vi "Create Measurement Client.vi"() -> ()   [LabVIEW 2021, in "MeasurementClient Editor.lvlib"]
uses:
  _MeasurementClient Utility/MeasurementClient Editor.lvlib
  <vilib>/Utility/error.llb/ErrWarn.ctl
  <vilib>/gRPC/Generated APIs/ni/measurementlink/discovery/v1/RPC Messages/ni_measurementlink_discovery_v1_EnumerateServicesRequest.ctl
  _Generator Helpers/Generator Helpers.lvlib
  <vilib>/gRPC/Generated APIs/ni/measurementlink/discovery/v1/ni.measurementlink.discovery.v1.api.lvlib
  <vilib>/Plug-In SDKs/Clients/Discovery V1/NI Discovery V1 Client.lvlib
panel:
  in  "Tab Control":enum32{"Inputs", "Status"}(tab)
  out "Active Project Name":string
  in  "Available Measurements":i32(listbox)=-1
  in  "Create Client":bool
  out "Warning":T1 caption="Measurement plug-in client name must be unique and cannot contain any of the following characters:\n           \\ / : * ? \" < > |"
  out "Error Message":string
  in  "Client Status":i32(listbox)=-1 caption="Measurement Plug-In Client Creation Status"
  # "* Project in which the measurement plug-in client vi will be created"
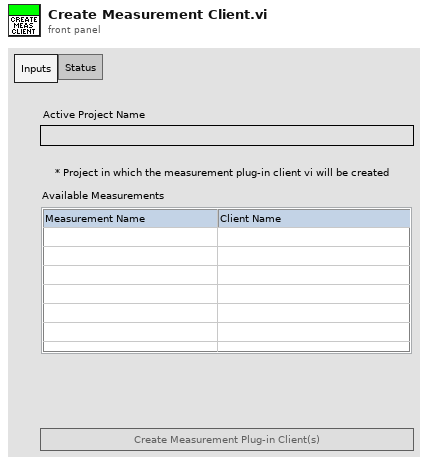
[diagram p1: front panel]
types:
  T1 = typedef "ErrWarn.ctl" = bool
  T2 = enum8{"Enabled", "Disabled", "Disabled and Grayed Out"}
  T3 = typedef "ni.measurementlink.discovery.v1.api.lvlib/ni_measurementlink_discovery_v1_EnumerateServicesRequest.ctl" = cluster{"provided_interface":string}
  T4 = typedef "ni.measurementlink.discovery.v1.api.lvlib/ni_measurementlink_discovery_v1_EnumerateServicesResponse.ctl" = cluster{"available_services":T5[]}
  T5 = typedef "ni.measurementlink.discovery.v1.api.lvlib/ni_measurementlink_discovery_v1_ServiceDescriptor.ctl" = cluster{"display_name":string, "description_url":string, "provided_interfaces":string[], "service_class":string, "annotations":T6[]}
  T6 = typedef "ni.measurementlink.discovery.v1.api.lvlib/ni_measurementlink_discovery_v1_ServiceDescriptor_AnnotationsEntry.ctl" = cluster{"key":string, "value":string}
  T7 = cluster{"project ref":refnum<vi>, "multicolumnListbox ref":refnum<vi>, "available measurement details":T4, "statusListbox ref":refnum<vi>, "error messages":string[]}
  T8 = typedef "ni.measurementlink.measurement.v2.api.lvlib/Measurement Service Client.lvlib/ni_measurementlink_measurement_v2_Output.ctl" = cluster{"field_number":i32, "type":T9, "name":string, "repeated":bool, "annotations":T10[], "message_type":string}
  T9 = typedef "ni.measurementlink.measurement.v2.api.lvlib/Measurement Service Client.lvlib/google_protobuf_Field_Kind.ctl" = enum32{"TYPE_UNKNOWN", "TYPE_DOUBLE", "TYPE_FLOAT", "TYPE_INT64", "TYPE_UINT64", "TYPE_INT32", "TYPE_FIXED64", "TYPE_FIXED32", "TYPE_BOOL", "TYPE_STRING", "TYPE_GROUP", "TYPE_MESSAGE", "TYPE_BYTES", "TYPE_UINT32", "TYPE_ENUM", "TYPE_SFIXED32", "TYPE_SFIXED64", "TYPE_SINT32", "TYPE_SINT64"}
  T10 = typedef "ni.measurementlink.measurement.v2.api.lvlib/Measurement Service Client.lvlib/ni_measurementlink_measurement_v2_Output_AnnotationsEntry.ctl" = cluster{"key":string, "value":string}
  T11 = typedef "ni.measurementlink.measurement.v2.api.lvlib/Measurement Service Client.lvlib/ni_measurementlink_measurement_v2_ConfigurationParameter.ctl" = cluster{"field_number":i32, "type":T9, "name":string, "repeated":bool, "annotations":T12[], "message_type":string}
  T12 = typedef "ni.measurementlink.measurement.v2.api.lvlib/Measurement Service Client.lvlib/ni_measurementlink_measurement_v2_ConfigurationParameter_AnnotationsEntry.ctl" = cluster{"key":string, "value":string}
  T13 = typedef "LVPoint32TypeDef.ctl" = cluster{"Horizontal":i32, "Vertical":i32}
  T14 = typedef "LVRowAndColumnTypeDef.ctl" = cluster{"Row":i32, "Column":i32}
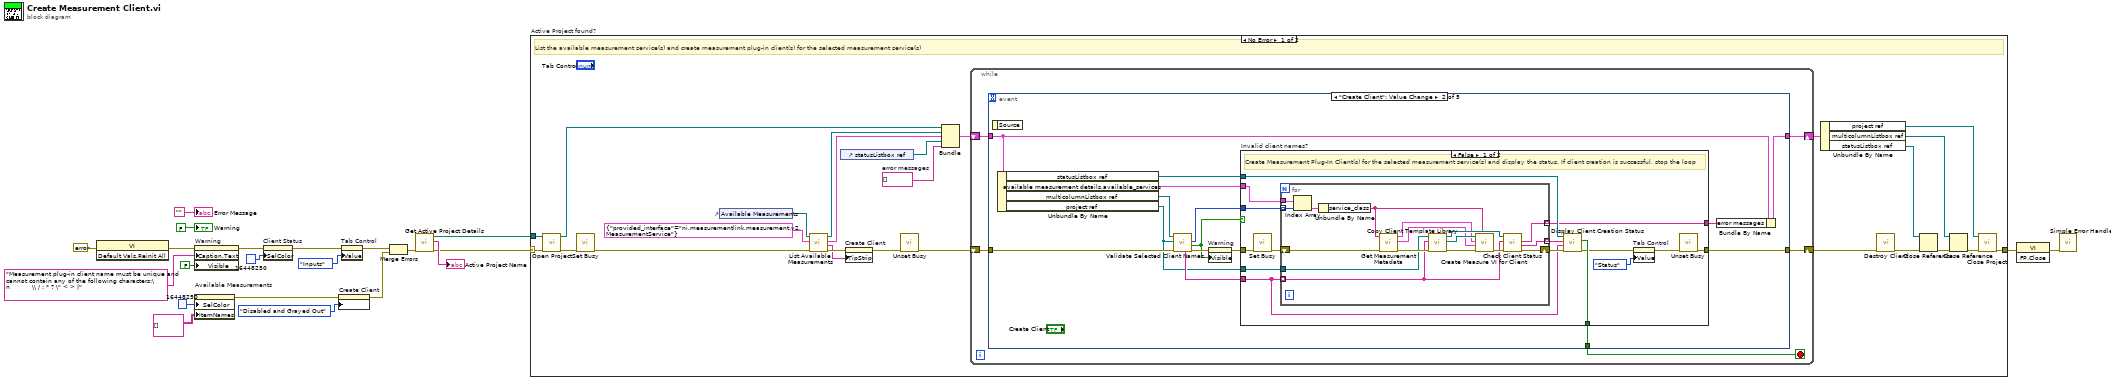
[diagram p0: block diagram]
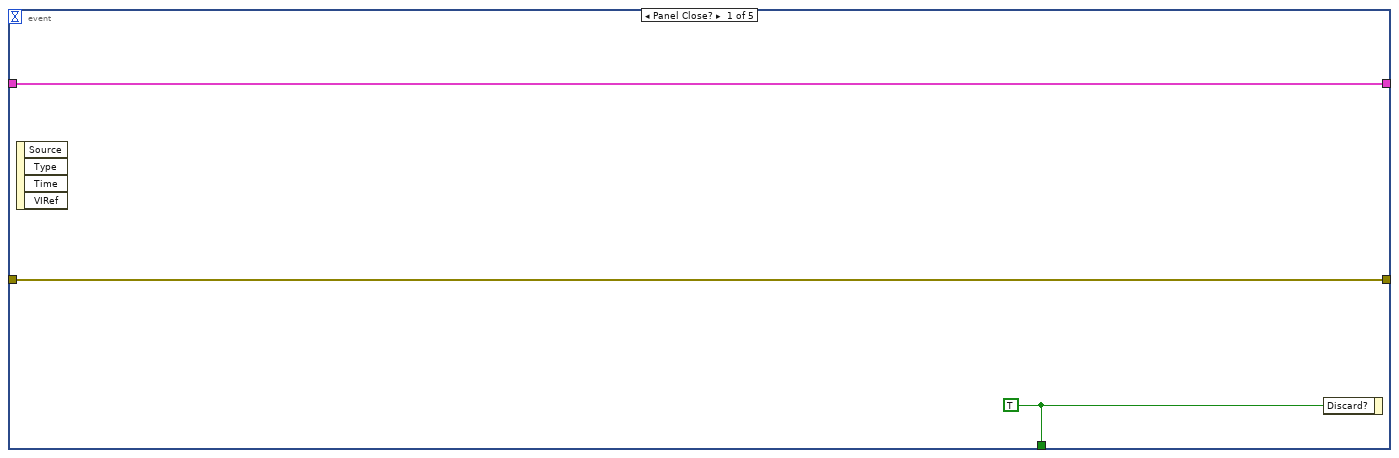
[diagram p2: hidden frame]
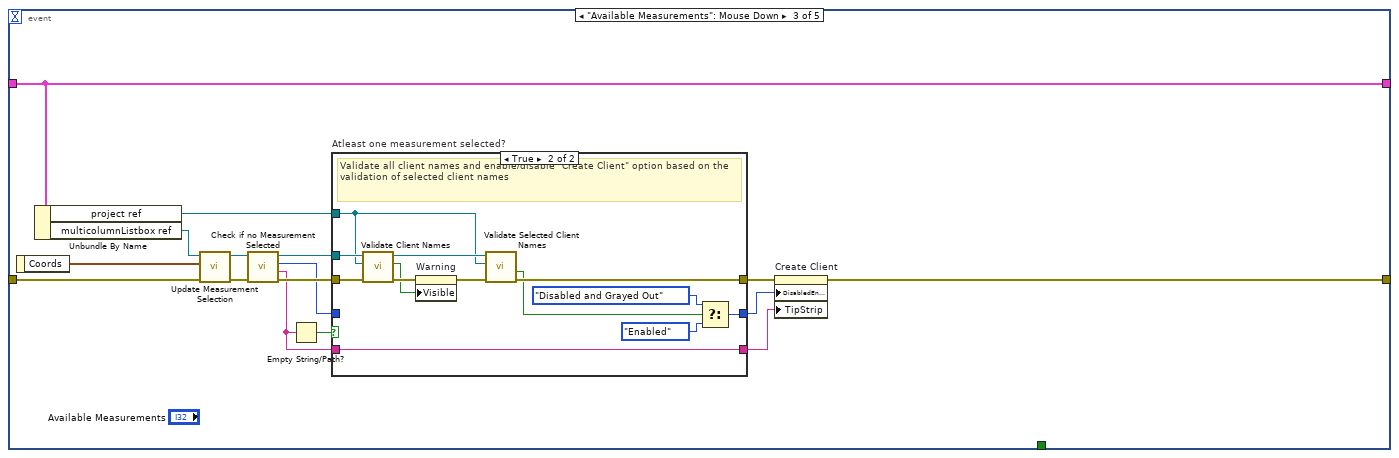
[diagram p4: hidden frame]
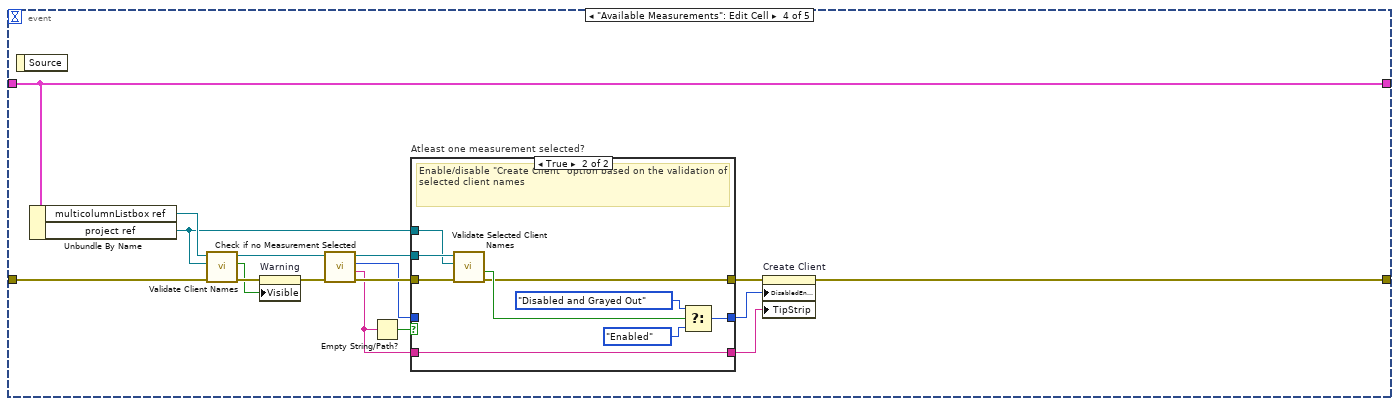
[diagram p6: hidden frame]
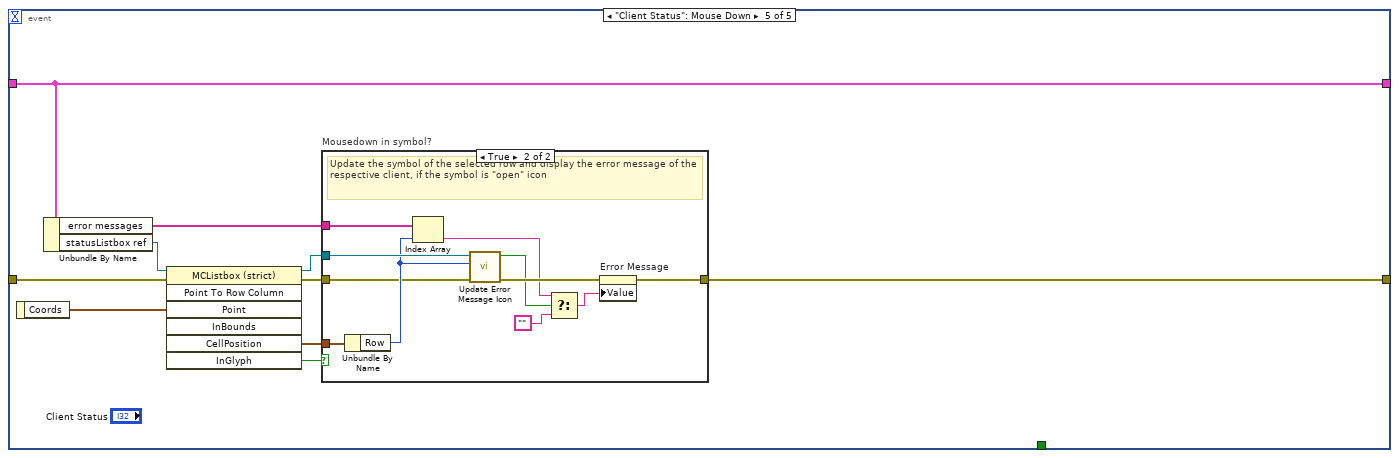
[diagram p8: hidden frame]
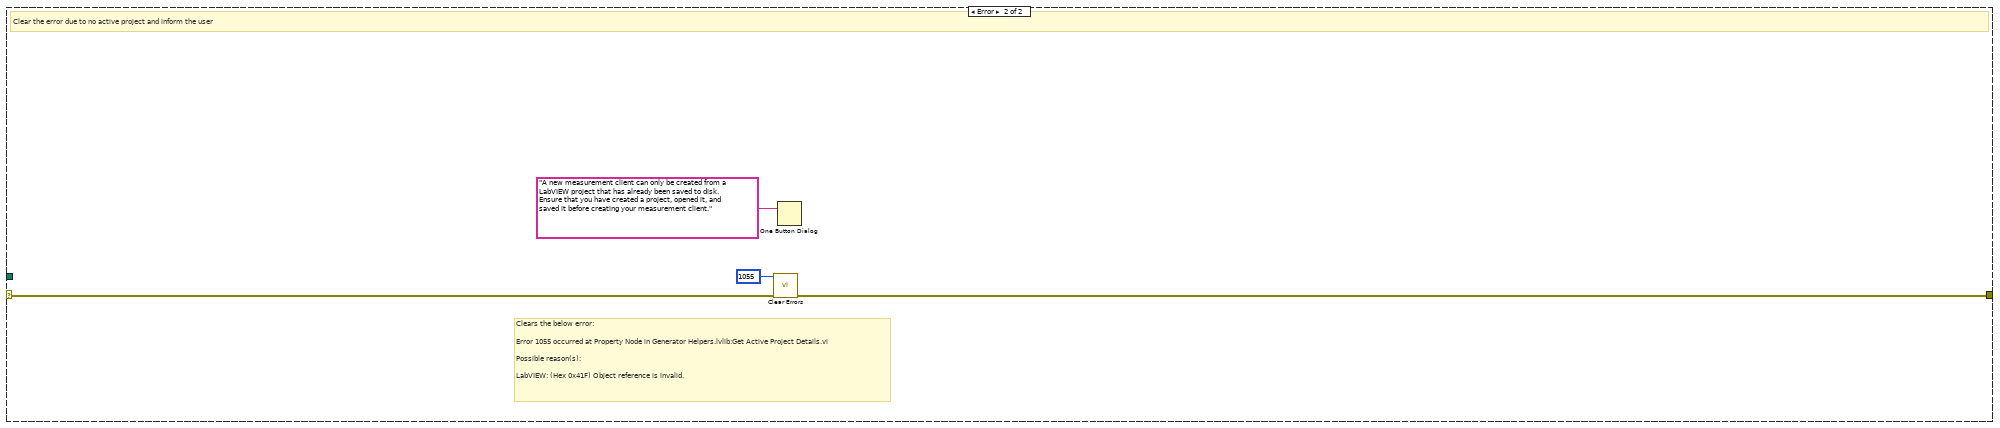
[diagram p10: hidden frame]
diagram:
  n1 = invoke class="VI" method="Default Vals.Reinit All"(error in=errorcluster {"status"=FALSE, "code"=0, "source"=""} ("error in (no error)")) -> (error out=w16:errorcluster)  [unwired: 2 in, 2 out]
  n2 = property on="Warning" class="Bool"(error in=w16, "Caption.Text"="Measurement plug-in client name must be unique and cannot contain any of the following characters:\n           \\ / : * ? \" < > |" ("Status"), "Visible"=FALSE) -> (error out=w6:errorcluster)  [unwired: 1 in, 1 out]
  n3 = property on="Available Measurements" class="MCListbox (strict)"("SelColor"=u32 16448250 ("Selection Color"), "ItemNames"=string[][] [] ("Item Names")) -> (error out=w3:errorcluster)  [unwired: 2 in, 1 out]
  n4 = property on="Client Status" class="MCListbox (strict)"(error in=w6, "SelColor"=u32 16448250 ("Selection Color")) -> (error out=w7:errorcluster)  [unwired: 1 in, 1 out]
  n5 = property on="Create Client" class="Bool"(error in=w3, "DisabledEnum"=T2."Disabled and Grayed Out" ("Disabled")) -> (error out=w2:errorcluster)  [unwired: 1 in, 1 out]
  n6 = property on="Tab Control" class="TabCtl (strict)"(error in=w7, "Value"=enum32{"Inputs", "Status"}."Inputs" ("Tab Control")) -> (error out=w5:errorcluster)  [unwired: 1 in, 1 out]
  n7 = Merge Errors(w5, w2) -> (w1:errorcluster)
  n8 = call "Get Active Project Details.vi"("error in"=w1) -> ("error out"=w11:errorcluster, "name"=→"Active Project Name":string, "path"=w15:path)  [unwired: 8 in]
  n9 = case "Active Project found?" shown="No Error" w11 {
    selector: w11 -> [w37 w187]
    tunnel: [w31 w190] -> w20
    tunnel: w15 -> [w47 _]
    frame No Error {
      w30 = string[] []  # error messages
      # "List the available measurement service(s) and create measurement plug-in client(s) for the selected measurement service(s)"
      n10 = call "Open Project.vi"("error in"=w37, "path"=w47) -> ("error out"=w38:errorcluster, "project ref"=w35:refnum<vi>)  [unwired: 8 in]
      n11 = call <vilib>:"Set Busy.vi"("error in (no error)"=w38) -> ("error out"=w40:errorcluster)  [unwired: 9 in, 1 out]
      n12 = control-ref of="Available Measurements"() -> (w43:refnum<vi>)
      n13 = call "List Available Measurements.vi"("error in (no error)"=w40, "enumerate services request"=T3 {"provided_interface"="ni.measurementlink.measurement.v2.MeasurementService"} ("request data"), "multicolumnListbox ref in"=w43) -> ("error out"=w42:errorcluster, "warning"=w24:string, "available measurement details"=w46:T4, "multicolumnListbox ref"=w27:refnum<vi>)  [unwired: 5 in]
      n14 = control-ref of="statusListbox ref"() -> (w23:refnum<vi>)
      n15 = property on="Create Client" class="Bool"(error in=w42, "TipStrip"=w24) -> (error out=w41:errorcluster)  [unwired: 1 in, 1 out]
      n16 = call <vilib>:"Unset Busy.vi"("error in (no error)"=w41) -> ("error out"=w39:errorcluster)  [unwired: 10 in]
      n17 = Bundle("project ref"=w35, "multicolumnListbox ref"=w27, "available measurement details"=w46, "statusListbox ref"=w23, "error messages"=w30) -> (w25:T7)  [unwired: 1 in]
      n18 = while {
        shift-right: [w51] -> w44
        shift-left: w39 -> [w52]
        shift-right: [w49] -> w26
        shift-left: w25 -> [w50]
        stop <- w48 stop-if-true
        n19 = event shown="[1] \"Create Client\": Value Change" {
          selector: _ -> [_ _ _ _ _]
          dyn-events: _ -> [_ _ _ _ _]
          timeout: _ -> [_ _ _ _ _]
          tunnel: w52 -> [w55 w70 w114 w151 w171]
          tunnel: [w55 w57 w113 w147 w174] -> w51
          tunnel: w50 -> [w54 w65 w119 w152 w172]
          tunnel: [w54 w61 w119 w152 w172] -> w49
          tunnel: [w53 w58 _ _ _] -> w48
          event Panel Close? {
            w53 = TRUE ("Discard?")
            # "Discard panel close and stop the execution of measurement plug-in client generator"
            n20 = event-data() -> ()  [unwired: 1 in, 4 out]
            n21 = event-data("Discard?"=w53) -> ()  [unwired: 1 in, 1 out]
          }
          event "Create Client": Value Change {
            # "Validate client name and create measurement plug-in client for the selected measurement service(s), if no invalid client name"
            n22 = event-data() -> ()  [unwired: 1 in, 1 out]
            n23 = Unbundle By Name(w65) -> ("statusListbox ref"=w62:refnum<vi>, "available measurement details.available_services"=w60:T5[], "multicolumnListbox ref"=w69:refnum<vi>, "project ref"=w63:refnum<vi>)
            n24 = call "Validate Selected Client Names.vi"("error in (no error)"=w70, "project ref"=w63, "multicolumnListbox in"=w69) -> ("error out"=w68:errorcluster, "warning?"=w59:bool, "selected measurement indices"=w66:i32[], "selected client names"=w64:string[])  [unwired: 4 in, 1 out]
            n25 = property on="Warning" class="Bool"(error in=w68, "Visible"=w59) -> (error out=w67:errorcluster)  [unwired: 1 in, 1 out]
            n26 = case "Invalid client names?" shown="False" w59 {
              tunnel: w67 -> [w85 w103]
              tunnel: w66 -> [w84 _]
              tunnel: w64 -> [w77 _]
              tunnel: w63 -> [w79 _]
              tunnel: [w72 w103] -> w57
              tunnel: w62 -> [w80 _]
              tunnel: w60 -> [w78 _]
              tunnel: [w76 _] -> w58
              tunnel: [w71 _] -> w56
              frame False {
                # "Create Measurement Plug-In Client(s) for the selected measurement service(s) and display the status. If client creation is successful, stop the loop"
                n27 = call <vilib>:"Set Busy.vi"("error in (no error)"=w85) -> ("error out"=w83:errorcluster)  [unwired: 9 in, 1 out]
                n28 = for {
                  tunnel: w78 -> [w100]
                  tunnel: w77 -> [w92] mode=indexing
                  shift-right: [w97] -> w82
                  shift-left: w83 -> [w94]
                  tunnel: w84 -> [w93] mode=indexing
                  tunnel: [w91] -> w81 mode=indexing
                  tunnel: w79 -> [w90]
                  tunnel: [w88] -> w71 mode=indexing
                  n29 = Index Array(array=w100, index=w93) -> (element=w99:T5)
                  n30 = Unbundle By Name(w99) -> ("service_class"=w89:string)
                  n31 = call "Get Measurement Metadata.vi"("error in"=w94, "service_class"=w89) -> ("error out"=w101:errorcluster, "outputs"=w86:T8[], "configuration_parameters"=w87:T11[])  [unwired: 7 in]
                  n32 = call "Copy Client Template Library.vi"("error in"=w101, "client name"=w92, "project ref"=w90) -> ("error out"=w102:errorcluster, "measure vi refnum"=w98:refnum<vi>, "project ref out"=w95:refnum<vi>)  [unwired: 6 in]
                  n33 = call "Create Measure VI for Client.vi"("client service_class"=w89, "error in"=w102, "results data"=w86, "configuration data"=w87, "measure vi refnum"=w98) -> ("error out"=w96:errorcluster)  [unwired: 6 in]
                  n34 = call "Check Client Status.vi"("error in"=w96, "client name"=w92, "project ref in"=w95) -> ("error out"=w97:errorcluster, "status"=w91:string, "error message"=w88:string)  [unwired: 5 in, 1 out]
                }
                n35 = call "Display Client Creation Status.vi"("error in"=w82, "client names"=w77, "status"=w81, "statusListbox in"=w80) -> ("error out"=w74:errorcluster, "all success?"=w76:bool)  [unwired: 5 in, 1 out]
                n36 = property on="Tab Control" class="TabCtl (strict)"(error in=w74, "Value"=enum32{"Inputs", "Status"}."Status" ("Tab Control")) -> (error out=w73:errorcluster)  [unwired: 1 in, 1 out]
                n37 = call <vilib>:"Unset Busy.vi"("error in (no error)"=w73) -> ("error out"=w72:errorcluster)  [unwired: 10 in]
              }
              frame True {
                # "Pass"
              }
            }
            n38 = Bundle By Name(cluster=w65, "error messages"=w56) -> (w61:T7)
          }
          event "Available Measurements": Mouse Down {
            # "Update the selection of measurement service and enable/disable \"Create Client\" accordingly"
            n39 = event-data() -> ("Coords"=w112:T13)  [unwired: 1 in]
            n40 = Unbundle By Name(w119) -> ("project ref"=w104:refnum<vi>, "multicolumnListbox ref"=w118:refnum<vi>)
            n41 = call "Update Measurement Selection.vi"("error in (no error)"=w114, "mouseDown coords"=w112, "multicolumnListbox in"=w118) -> ("error out"=w116:errorcluster, "multicolumnListbox out"=w117:refnum<vi>)  [unwired: 7 in]
            n42 = call "Check if no Measurement Selected.vi"("error in (no error)"=w116, "multicolumnListbox in"=w117) -> ("error out"=w115:errorcluster, "warning?"=w105:string, "create client disabled?"=w107:T2, "multicolumnListbox out"=w110:refnum<vi>)  [unwired: 6 in]
            n43 = Empty String/Path?(string/path=w105) -> (empty?=w109:bool)
            n44 = case "Atleast one measurement selected?" shown="True" w109 {
              tunnel: w115 -> [w122 w127]
              tunnel: [w122 w131] -> w111
              tunnel: w110 -> [_ w126]
              tunnel: [w121 w132] -> w106
              tunnel: w105 -> [w121 w132]
              tunnel: [w120 w133] -> w108
              tunnel: w107 -> [w120 _]
              tunnel: w104 -> [_ w123]
              frame False {
                # "Enable/disable the \"Create Client\" option based on measurement selection"
              }
              frame True {
                # "Validate all client names and enable/disable \"Create Client\" option based on the validation of selected client names"
                n45 = call "Validate Client Names.vi"("error in (no error)"=w127, "project ref"=w123, "multicolumnListbox in"=w126) -> ("error out"=w129:errorcluster, "warning?"=w128:bool, "multicolumnListbox out"=w125:refnum<vi>)  [unwired: 6 in]
                n46 = property on="Warning" class="Bool"(error in=w129, "Visible"=w128) -> (error out=w124:errorcluster)  [unwired: 1 in, 1 out]
                n47 = call "Validate Selected Client Names.vi"("error in (no error)"=w124, "project ref"=w123, "multicolumnListbox in"=w125) -> ("error out"=w131:errorcluster, "warning?"=w130:bool)  [unwired: 4 in, 3 out]
                n48 = Select(t=T2."Disabled and Grayed Out" ("Disabled"), s=w130, f=T2."Enabled") -> (s? t:f=w133:T2)
              }
            }
            n49 = property on="Create Client" class="Bool"(error in=w111, "DisabledEnum"=w108, "TipStrip"=w106) -> (error out=w113:errorcluster)  [unwired: 1 in, 1 out]
          }
          event "Available Measurements": Edit Cell {
            n50 = event-data() -> ()  [unwired: 1 in, 1 out]
            n51 = Unbundle By Name(w152) -> ("multicolumnListbox ref"=w148:refnum<vi>, "project ref"=w136:refnum<vi>)
            n52 = call "Validate Client Names.vi"("error in (no error)"=w151, "project ref"=w136, "multicolumnListbox in"=w148) -> ("error out"=w150:errorcluster, "warning?"=w149:bool, "multicolumnListbox out"=w143:refnum<vi>)  [unwired: 6 in]
            n53 = property on="Warning" class="Bool"(error in=w150, "Visible"=w149) -> (error out=w144:errorcluster)  [unwired: 1 in, 1 out]
            n54 = call "Check if no Measurement Selected.vi"("error in (no error)"=w144, "multicolumnListbox in"=w143) -> ("error out"=w141:errorcluster, "warning?"=w137:string, "create client disabled?"=w139:T2, "multicolumnListbox out"=w142:refnum<vi>)  [unwired: 6 in]
            n55 = Empty String/Path?(string/path=w137) -> (empty?=w140:bool)
            n56 = case "Atleast one measurement selected?" shown="True" w140 {
              tunnel: [w154 w163] -> w146
              tunnel: [w155 w160] -> w145
              tunnel: w142 -> [_ w159]
              tunnel: w141 -> [w154 w158]
              tunnel: w139 -> [w155 _]
              tunnel: [w153 w157] -> w138
              tunnel: w137 -> [w153 w157]
              tunnel: w136 -> [_ w156]
              frame False {
                # "Enable/disable the \"Create Client\" option based on measurement selection"
              }
              frame True {
                # "Enable/disable \"Create Client\" option based on the validation of selected client names"
                n57 = call "Validate Selected Client Names.vi"("error in (no error)"=w158, "project ref"=w156, "multicolumnListbox in"=w159) -> ("error out"=w163:errorcluster, "warning?"=w164:bool)  [unwired: 4 in, 3 out]
                n58 = Select(t=T2."Disabled and Grayed Out" ("Disabled"), s=w164, f=T2."Enabled") -> (s? t:f=w160:T2)
              }
            }
            n59 = property on="Create Client" class="Bool"(error in=w146, "DisabledEnum"=w145, "TipStrip"=w138) -> (error out=w147:errorcluster)  [unwired: 1 in, 1 out]
          }
          event "Client Status": Mouse Down {
            n60 = event-data() -> ("Coords"=w168:T13)  [unwired: 1 in]
            n61 = Unbundle By Name(w172) -> ("error messages"=w173:string[], "statusListbox ref"=w169:refnum<vi>)
            n62 = invoke class="MCListbox (strict)" method="Point To Row Column"(reference=w169, error in=w171, "Point"=w168) -> (reference out=w166:refnum<vi>, error out=w170:errorcluster, "CellPosition"=w167:T14, "InGlyph"=w165:bool)  [unwired: 4 in, 3 out]
            n63 = case "Mousedown in symbol?" shown="True" w165 {
              tunnel: [w175 w180] -> w174
              tunnel: w167 -> [_ w186]
              tunnel: w173 -> [_ w185]
              tunnel: w170 -> [w175 w182]
              tunnel: w166 -> [_ w184]
              frame False {
                # "Pass"
              }
              frame True {
                # "Update the symbol of the selected row and display the error message of the respective client, if the symbol is \"open\" icon"
                n64 = Unbundle By Name(w186) -> ("Row"=w183:i32)
                n65 = Index Array(array=w185, index=w183) -> (element=w178:string)
                n66 = call "Update Error Message Icon.vi"("error in"=w182, "selected row"=w183, "statusListbox in"=w184) -> ("error out"=w181:errorcluster, "open?"=w179:bool)  [unwired: 7 in]
                n67 = Select(t=w178, s=w179, f="") -> (s? t:f=w176:string)
                n68 = property on="Error Message" class="Str"(error in=w181, "Value"=w176) -> (error out=w180:errorcluster)  [unwired: 1 in, 1 out]
              }
            }
          }
        }
      }
      n69 = Unbundle By Name(w26) -> ("project ref"=w32:refnum<vi>, "multicolumnListbox ref"=w45:refnum<vi>, "statusListbox ref"=w28:refnum<vi>)
      n70 = call <vilib>:"Destroy Client.vi"("error in"=w44) -> ("error out"=w34:errorcluster)  [unwired: 10 in]
      n71 = Close Reference(reference=w28, error in (no error)=w34) -> (error out=w29:errorcluster)
      n72 = Close Reference(reference=w45, error in (no error)=w29) -> (error out=w33:errorcluster)
      n73 = call "Close Project.vi"("error in"=w33, "project ref"=w32) -> ("error out"=w31:errorcluster)  [unwired: 9 in]
    }
    frame Error {
      # "Clears the below error:\n\nError 1055 occurred at Property Node in Generator Helpers.lvlib:Get Active Project Details.vi\n\nPossible reason(s):\n\nLabVIEW: (Hex 0x41F) Object reference is invalid."
      # "Clear the error due to no active project and inform the user"
      n74 = call <vilib>:"Clear Errors.vi"("error in (no error)"=w187, "specific error code to clear (0: all)"=1055) -> ("error out"=w190:errorcluster)  [unwired: 4 in, 1 out]
      n75 = One Button Dialog(message="A new measurement client can only be created from a LabVIEW project that has already been saved to disk.  Ensure that you have created a project, opened it, and saved it before creating your measurement client.") -> ()  [unwired: 1 in, 1 out]
    }
  }
  n76 = invoke class="VI" method="FP.Close"(error in=w20) -> (error out=w22:errorcluster)  [unwired: 2 in, 2 out]
  n77 = call <vilib>:"Simple Error Handler.vi"("error in (no error)"=w22) -> ()  [unwired: 4 in, 5 out]
  "Warning" <- T1 FALSE ("Warning")
  "Error Message" <- ""
